vi "Format Number to V or mV.vi"(8 "error in (no error)":errorcluster, 11 "Value":dbl) -> (0 "error out":errorcluster, 1 "Units":string, 2 "Value Out":string, 3 "Value Out (DBL)":dbl)   [LabVIEW 2018]
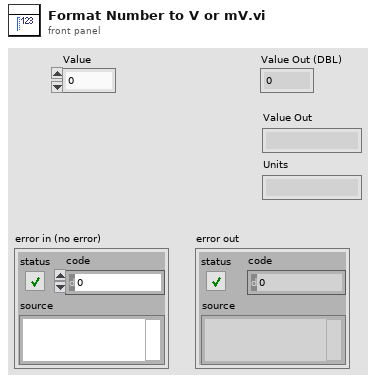
[diagram p1: front panel]
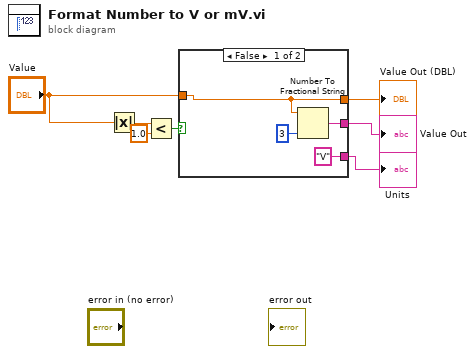
[diagram p0: block diagram]
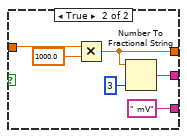
[diagram p2: hidden frame]
diagram:
  n1 = Absolute Value(x="Value") -> (abs(x)=w7:dbl)
  n2 = Less?(x=w7, y=1.0) -> (x < y?=w5:bool)
  n3 = case shown="False" w5 {
    tunnel: "Value" -> [w9 w17]
    tunnel: [w9 w15] -> w3
    tunnel: [w10 w13] -> w2
    tunnel: ["V" " mV"] -> w1
    frame False {
      n4 = Number To Fractional String(number=w9, precision (6)=i16 3) -> (F-format string=w10:string)  [unwired: 2 in]
    }
    frame True {
      n5 = Multiply(x=w17, y=1000.0) -> (x*y=w15:dbl)
      n6 = Number To Fractional String(number=w15, precision (6)=i16 3) -> (F-format string=w13:string)  [unwired: 2 in]
    }
  }
  "Value Out" <- w2
  "Value Out (DBL)" <- w3
  "Units" <- w1
